vi "MGI Get Parent Directory.vi"(8 "Error In":errorcluster, 11 "VI Reference (Top Level)":refnum<vi>) -> (0 "Error Out":errorcluster, 3 "Parent Directory":path)   [LabVIEW 2020]
doc: "If this VI is called from the LabVIEW Development environment, it outputs the file directory containing the specified vi. If the VI is inside an llb, then the directory containing the llb is output.\nIf this VI is called from a built executable, it outputs the file directory containing the built executable.\n\nAuthored by Matthew Harrison\nsupport@mooregoodideas.com\nwww.mooregoodideas.com\n\nCopyright (c) 2010, Moore Good Ideas, Inc.\n\nAll rights reserved.\n\nRedistribution and use in source and binary forms, with or without modification, are permitted provided that the following conditions are met:\n\n * Redistributions of source code must retain the above copyright notice, this list of conditions and the following disclaimer.\n * Redistributions in binary form must reproduce the above copyright notice, this list of conditions and the following disclaimer in the documentation and/or other materials provided with the distribution.\n * Neither the name of Moore Good Ideas, Inc. nor the names of its contributors may be used to endorse or promote products derived from this software without specific prior written permission.\n\nTHIS SOFTWARE IS PROVIDED BY THE COPYRIGHT HOLDERS AND CONTRIBUTORS \"AS IS\" AND ANY EXPRESS OR IMPLIED WARRANTIES, INCLUDING, BUT NOT LIMITED TO, THE IMPLIED WARRANTIES OF MERCHANTABILITY AND FITNESS FOR A PARTICULAR PURPOSE ARE DISCLAIMED. IN NO EVENT SHALL THE COPYRIGHT OWNER OR CONTRIBUTORS BE LIABLE FOR ANY DIRECT, INDIRECT, INCIDENTAL, SPECIAL, EXEMPLARY, OR CONSEQUENTIAL DAMAGES (INCLUDING, BUT NOT LIMITED TO, PROCUREMENT OF SUBSTITUTE GOODS OR SERVICES; LOSS OF USE, DATA, OR PROFITS; OR BUSINESS INTERRUPTION) HOWEVER CAUSED AND ON ANY THEORY OF LIABILITY, WHETHER IN CONTRACT, STRICT LIABILITY, OR TORT (INCLUDING NEGLIGENCE OR OTHERWISE) ARISING IN ANY WAY OUT OF THE USE OF THIS SOFTWARE, EVEN IF ADVISED OF THE POSSIBILITY OF SUCH DAMAGE."
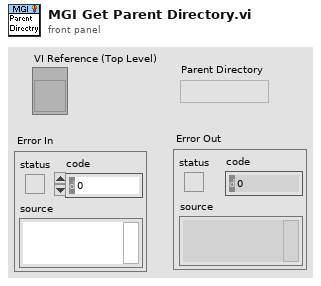
[diagram p1: front panel]
types:
  T1 = enum32{"invalid app kind", "Development System", "Run Time System", "Student Edition", "Embedded LabVIEW", "Evaluation", "Custom"}
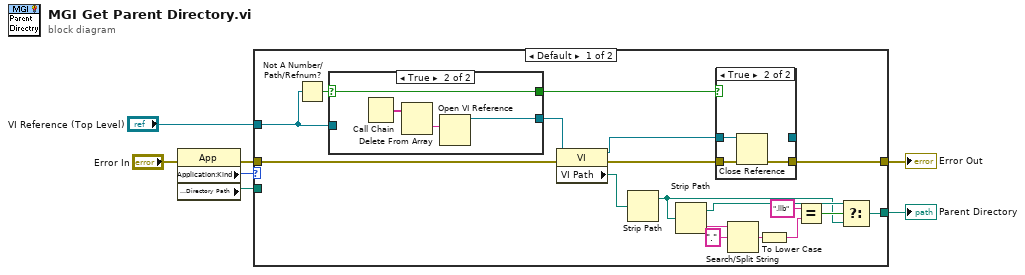
[diagram p0: block diagram]
diagram:
  n1 = property class="App"(error in="Error In") -> (error out=w4:errorcluster, "Application:Kind"=w7:T1, "Application:Directory Path"=w6:path)  [unwired: 1 in, 1 out]
  n2 = case shown="Default" w7 {
    tunnel: w6 -> [_ w37]
    tunnel: [w16 w37] -> w2
    tunnel: w4 -> [w13 w36]
    tunnel: [w8 w36] -> w3
    tunnel: "VI Reference (Top Level)" -> [w14 _]
    frame Default {
      n3 = Not A Number/Path/Refnum?(number/path/refnum=w14) -> (NaN/Path/Refnum?=w15:bool)
      n4 = case shown="True" w15 {
        selector: w15 -> [_ w35]
        tunnel: [w31 w32] -> w12
        tunnel: w14 -> [w31 _]
        tunnel: [_ w35] -> w11
        frame False {
        }
        frame True {
          n5 = Call Chain() -> (call chain=w33:string[])
          n6 = Delete From Array(array=w33) -> (deleted portion=w34:string)  [unwired: 2 in, 1 out]
          n7 = Open VI Reference(vi path=w34) -> (vi reference=w32:refnum<vi>)  [unwired: 5 in, 1 out]
        }
      }
      n8 = property class="VI"(reference=w12, error in=w13) -> (reference out=w9:refnum<vi>, error out=w10:errorcluster, "VI Path"=w25:path)
      n9 = Strip Path(path=w25) -> (stripped path=w17:path)  [unwired: 1 out]
      n10 = Strip Path(path=w17) -> (stripped path=w18:path, name=w24:string)
      n11 = case shown="True" w11 {
        tunnel: w9 -> [w26 w30]
        tunnel: w10 -> [w27 w29]
        tunnel: [w27 w28] -> w8
        tunnel: [w26 _] -> _
        frame False {
        }
        frame True {
          n12 = Close Reference(reference=w30, error in (no error)=w29) -> (error out=w28:errorcluster)
        }
      }
      n13 = Search/Split String(string=w24, search string/char (-)="." ("search char (-)")) -> (match + rest of string=w22:string)  [unwired: 1 in, 2 out]
      n14 = To Lower Case(string=w22) -> (all lower case string=w21:string)
      n15 = Equal?(x=".llb", y=w21) -> (x = y?=w19:bool)
      n16 = Select(t=w18, s=w19, f=w17) -> (s? t:f=w16:path)
    }
    frame "Run Time System", "Embedded LabVIEW" {
    }
  }
  "Parent Directory" <- w2
  "Error Out" <- w3
